vi "KE622x -- 2182 -A Get Params.vi"(0 "622x Resource In":refnum<visa-resource-name>, 1 "Check For SCPI Errors? (T)":bool=TRUE, 11 "error in (no error)":errorcluster) -> (4 "622x Resource Out (dupl)":refnum<visa-resource-name>, 8 "2812 -A Params":T6={"Auto Range?"=FALSE, "Man / Selected\nRange"=enum."10mV", "Enable Digital\nFilter?"=FALSE, "Filter Type"=enum."Moving", "Filter Count"=10, "Filter\nWindow (%)"=0.01, "Enable Analog\nFilter?"=FALSE, "NPLCs"=5} {"Filter\nWindow (%)" min=0.0 max=10.0 step=0.01 format="%.2f"; "Filter Count" min=1 max=100; "NPLCs" min=1 max=60}, 15 "error out":errorcluster)   [LabVIEW 2019, in "Keithley 622x.lvlib"]
doc: "Returns the measurement parameters for the 2182/2182A connected to the 622x via the RS232 link."
uses:
  Keithley 622x.lvlib
  Low Level/Typedefs/KE2182 -- Voltage Ranges.ctl
  Low Level/Typedefs/KE2182 -- Filter Type.ctl
  Low Level/Typedefs/KE2182 -- Filter Count.ctl
  Low Level/Typedefs/KE2182 -- Filter Window.ctl
  Low Level/Typedefs/KE2182 -- NPLCs.ctl
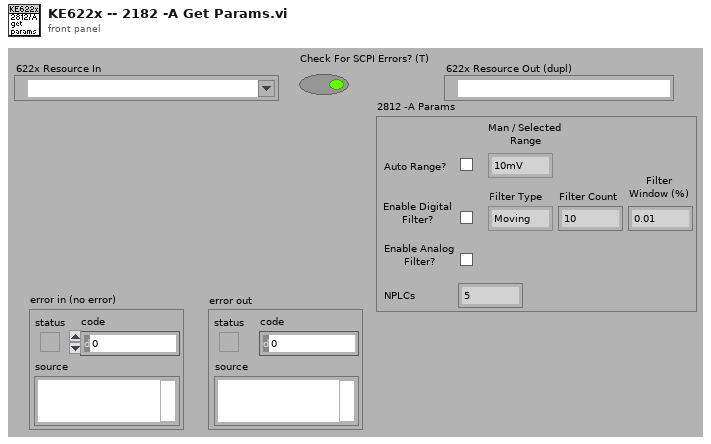
[diagram p1: front panel]
types:
  T1 = typedef "Keithley 622x.lvlib/KE2182 -- Voltage Ranges.ctl" = enum16{"10mV", "100mV", "1V", "10V", "100V"}
  T2 = typedef "Keithley 622x.lvlib/KE2182 -- Filter Type.ctl" = enum16{"Moving", "Repeat"}
  T3 = typedef "Keithley 622x.lvlib/KE2182 -- Filter Count.ctl" = u32
  T4 = typedef "Keithley 622x.lvlib/KE2182 -- Filter Window.ctl" = dbl
  T5 = typedef "Keithley 622x.lvlib/KE2182 -- NPLCs.ctl" = u32
  T6 = cluster{"Auto Range?":bool, "Man / Selected\nRange":T1, "Enable Digital\nFilter?":bool, "Filter Type":T2, "Filter Count":T3, "Filter\nWindow (%)":T4, "Enable Analog\nFilter?":bool, "NPLCs":T5}
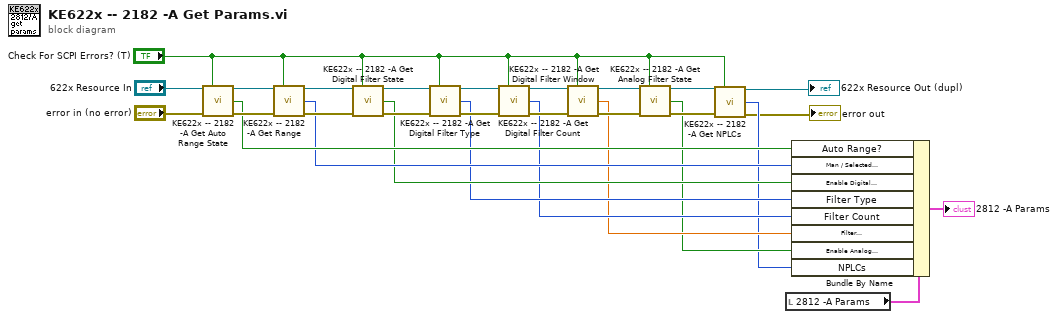
[diagram p0: block diagram]
diagram:
  n1 = call "KE622x -- 2182 -A Get Auto Range State.vi"("622x Resource In"="622x Resource In", "Check For SCPI Errors? (T)"="Check For SCPI Errors? (T)", "error in (no error)"="error in (no error)") -> ("622x Resource Out (dupl)"=w26:refnum<visa-resource-name>, "Auto Range Enabled?"=w15:bool, "error out"=w25:errorcluster)  [unwired: 10 in]
  n2 = call "KE622x -- 2182 -A Get Range.vi"("622x Resource In"=w26, "Check For SCPI Errors? (T)"="Check For SCPI Errors? (T)", "error in (no error)"=w25) -> ("622x Resource Out (dupl)"=w24:refnum<visa-resource-name>, "2182/2182A Range"=w14:T1, "error out"=w23:errorcluster)  [unwired: 10 in]
  n3 = call "KE622x -- 2182 -A Get Digital Filter State.vi"("622x Resource In"=w24, "Check For SCPI Errors? (T)"="Check For SCPI Errors? (T)", "error in (no error)"=w23) -> ("622x Resource Out (dupl)"=w22:refnum<visa-resource-name>, "Digital Filter Enabled?"=w13:bool, "error out"=w21:errorcluster)  [unwired: 10 in]
  n4 = call "KE622x -- 2182 -A Get Digital Filter Type.vi"("622x Resource In"=w22, "Check For SCPI Errors? (T)"="Check For SCPI Errors? (T)", "error in (no error)"=w21) -> ("622x Resource Out (dupl)"=w20:refnum<visa-resource-name>, "Filter Type"=w12:T2, "error out"=w19:errorcluster)  [unwired: 10 in]
  n5 = call "KE622x -- 2182 -A Get Digital Filter Count.vi"("622x Resource In"=w20, "Check For SCPI Errors? (T)"="Check For SCPI Errors? (T)", "error in (no error)"=w19) -> ("622x Resource Out (dupl)"=w7:refnum<visa-resource-name>, "Filter Count"=w11:T3, "error out"=w18:errorcluster)  [unwired: 10 in]
  n6 = call "KE622x -- 2182 -A Get Digital Filter Window.vi"("622x Resource In"=w7, "Check For SCPI Errors? (T)"="Check For SCPI Errors? (T)", "error in (no error)"=w18) -> ("622x Resource Out (dupl)"=w6:refnum<visa-resource-name>, "Filter Window (%)"=w10:T4, "error out"=w17:errorcluster)  [unwired: 10 in]
  n7 = call "KE622x -- 2182 -A Get Analog Filter State.vi"("622x Resource In"=w6, "Check For SCPI Errors? (T)"="Check For SCPI Errors? (T)", "error in (no error)"=w17) -> ("622x Resource Out (dupl)"=w5:refnum<visa-resource-name>, "Analog Filter Enabled?"=w9:bool, "error out"=w16:errorcluster)  [unwired: 10 in]
  n8 = call "KE622x -- 2182 -A Get NPLCs.vi"("622x Resource In"=w5, "Check For SCPI Errors? (T)"="Check For SCPI Errors? (T)", "error in (no error)"=w16) -> ("622x Resource Out (dupl)"=→"622x Resource Out (dupl)":refnum<visa-resource-name>, "2182 -A NPLCs"=w8:T5, "error out"=→"error out":errorcluster)  [unwired: 10 in]
  n9 = local read "2812 -A Params"() -> (w29:T6)
  n10 = Bundle By Name(cluster=w29, "Auto Range?"=w15, "Man / Selected\nRange"=w14, "Enable Digital\nFilter?"=w13, "Filter Type"=w12, "Filter Count"=w11, "Filter\nWindow (%)"=w10, "Enable Analog\nFilter?"=w9, "NPLCs"=w8) -> (→"2812 -A Params":T6)
